vi "Decrement by One.vi"(9 "Schedule Cell in":refnum<class "Schedule Cell.lvclass">) -> (3 "Schedule Cell out":refnum<class "Schedule Cell.lvclass">, 4 "Last Script":bool)   [LabVIEW 2020, in "TALOS.lvlib" / "Run Utilities.lvlib" / "Schedule Cell.lvclass"]
doc: "Decrement the number of repetitions by 1."
uses:
  Schedule Cell.lvclass
  Schedule Cell.lvclass/Schedule Cell.ctl
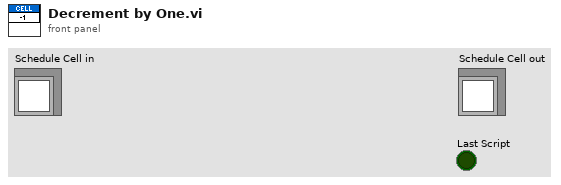
[diagram p1: front panel]
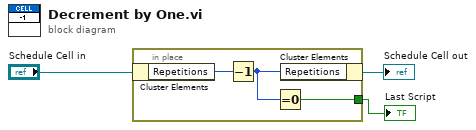
[diagram p0: block diagram]
diagram:
  n1 = in-place {
    in-place-border: [w4] -> w1
    n2 = in-place-cluster #1("Schedule Cell in") -> ("Repetitions"=w6:u32)
    n3 = Decrement(x=w6) -> (x-1=w5:u32)
    n4 = Equal To 0?(x=w5) -> (x = 0?=w4:bool)
    n5 = in-place-cluster #1("Repetitions"=w5) -> (→"Schedule Cell out":refnum<class "Schedule Cell.lvclass">)
  }
  "Last Script" <- w1
